vi "advanced_settings.vi"(0 "input cluster":T3) -> (1 "Output AFG resource name":refnum<k15>, 2 "Set?":bool)   [LabVIEW 2010]
uses:
  <vilib>/vision/Avi1.llb/AviRefnum.ctl
  <vilib>/userDefined/High Color/IMAQdx.ctl
panel:
  in  "Use Background Division Image Correction?":bool=TRUE
  in  "Aggregate Output?":bool
  in  "Number of Image Adaptation Bands":i32=10 step=1
  in  "stop":bool
  in  "OK Button":bool
  in  "AFG resource name":refnum<k15>="COM1"
  in  "Object Border":i32=20
  in  "Frames of Adaptation":i32=10
  in  "Bit Depth from Camera?":bool=TRUE
  in  "Image Bit Depth":u32=12
  in  "Adaptation Rate":i32=5 step=1
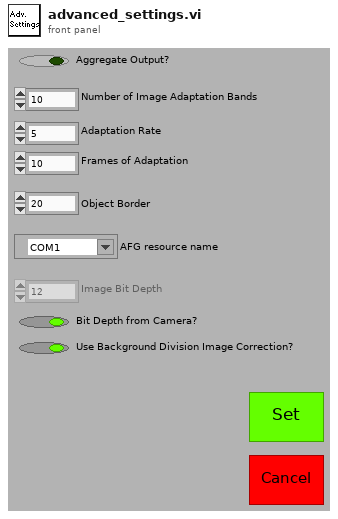
[diagram p1: front panel]
types:
  T1 = typedef "AviRefnum.ctl" = refnum<k1>
  T2 = typedef "IMAQdx.ctl" = refnum<k21>
  T3 = cluster{cluster{"Path":refnum<vi>, "Prefix":refnum<vi>, "Type of object to track":refnum<vi>, "Object Contrast (%)":refnum<vi>, "Fill Hysteresis (%)":refnum<vi>, "Maximum Object Size (pixels)":refnum<vi>, "Minimum Object Size (pixels)":refnum<vi>, "Object Size hysteresis (%)":refnum<vi>, "Image Binning":refnum<vi>, "Contour?":refnum<vi>, "Skeletonize?":refnum<vi>, "Frames of Adaptation":refnum<vi>, "Adaptation Rate":refnum<vi>, "Object Border":refnum<vi>, "Image Bit Depth":refnum<vi>, "Bit Depth from Camera?":refnum<vi>, "AFG resource name":refnum<vi>, "IMAQ Camera Interface Name":refnum<vi>, "Device auto-start delay (s)":refnum<vi>, "Number of Image Adaptation Bands":refnum<vi>, "Experiment Duration (s)":refnum<vi>, "Tap":refnum<vi>, "Tap Delay":refnum<vi>, "Tap Interval":refnum<vi>, "Tap Number":refnum<vi>, "Tap Stimulus Method":refnum<vi>, "Advanced Tap Settings":refnum<vi>, "Puff":refnum<vi>, "Puff Delay":refnum<vi>, "Puff Interval":refnum<vi>, "Puff Number":refnum<vi>, "Puff Stimulus Method":refnum<vi>, "Advanced Puff Settings":refnum<vi>, "Custom 1":refnum<vi>, "Custom 1 Delay":refnum<vi>, "Custom 1 Interval":refnum<vi>, "Custom 1 Number":refnum<vi>, "Custom 1 Stimulus Method":refnum<vi>, "Advanced Custom 1 Settings":refnum<vi>, "puff fraction of time between is active":refnum<vi>, "time between puff onset":refnum<vi>, "tap fraction of time between is active":refnum<vi>, "time between tap onset":refnum<vi>, "Tap Train Number":refnum<vi>, "custom 1 fraction of time between is active":refnum<vi>, "time between custom 1 onset":refnum<vi>, "Custom 2":refnum<vi>, "Custom 2 Delay":refnum<vi>, "Custom 2 Interval":refnum<vi>, "Custom 2 Number":refnum<vi>, "Custom 2 Stimulus Method":refnum<vi>, "Advanced Custom 2 Settings":refnum<vi>, "custom 2 fraction of time between is active":refnum<vi>, "time between custom 2 onset":refnum<vi>, "Save":refnum<vi>, "Load":refnum<vi>, "Raw Image Save Interval (s)":refnum<vi>, "Turn on output aggregation?":refnum<vi>, "Turn on Background division algorithm":refnum<vi>, "Turn on external triggering of camera":refnum<vi>}, cluster{"IMAQ Session Out":refnum<k11>, "Avi Refnum":T1, "Value":enum32{"IMAQ interface", "IMAQdx interface", "AVI file"}, "Value":T2, "Value":bool}}
  T4 = cluster{"Path":refnum<vi>, "Prefix":refnum<vi>, "Type of object to track":refnum<vi>, "Object Contrast (%)":refnum<vi>, "Fill Hysteresis (%)":refnum<vi>, "Maximum Object Size (pixels)":refnum<vi>, "Minimum Object Size (pixels)":refnum<vi>, "Object Size hysteresis (%)":refnum<vi>, "Image Binning":refnum<vi>, "Contour?":refnum<vi>, "Skeletonize?":refnum<vi>, "Frames of Adaptation":refnum<vi>, "Adaptation Rate":refnum<vi>, "Object Border":refnum<vi>, "Image Bit Depth":refnum<vi>, "Bit Depth from Camera?":refnum<vi>, "AFG resource name":refnum<vi>, "IMAQ Camera Interface Name":refnum<vi>, "Device auto-start delay (s)":refnum<vi>, "Number of Image Adaptation Bands":refnum<vi>, "Experiment Duration (s)":refnum<vi>, "Tap":refnum<vi>, "Tap Delay":refnum<vi>, "Tap Interval":refnum<vi>, "Tap Number":refnum<vi>, "Tap Stimulus Method":refnum<vi>, "Advanced Tap Settings":refnum<vi>, "Puff":refnum<vi>, "Puff Delay":refnum<vi>, "Puff Interval":refnum<vi>, "Puff Number":refnum<vi>, "Puff Stimulus Method":refnum<vi>, "Advanced Puff Settings":refnum<vi>, "Custom 1":refnum<vi>, "Custom 1 Delay":refnum<vi>, "Custom 1 Interval":refnum<vi>, "Custom 1 Number":refnum<vi>, "Custom 1 Stimulus Method":refnum<vi>, "Advanced Custom 1 Settings":refnum<vi>, "puff fraction of time between is active":refnum<vi>, "time between puff onset":refnum<vi>, "tap fraction of time between is active":refnum<vi>, "time between tap onset":refnum<vi>, "Tap Train Number":refnum<vi>, "custom 1 fraction of time between is active":refnum<vi>, "time between custom 1 onset":refnum<vi>, "Custom 2":refnum<vi>, "Custom 2 Delay":refnum<vi>, "Custom 2 Interval":refnum<vi>, "Custom 2 Number":refnum<vi>, "Custom 2 Stimulus Method":refnum<vi>, "Advanced Custom 2 Settings":refnum<vi>, "custom 2 fraction of time between is active":refnum<vi>, "time between custom 2 onset":refnum<vi>, "Save":refnum<vi>, "Load":refnum<vi>, "Raw Image Save Interval (s)":refnum<vi>, "Turn on output aggregation?":refnum<vi>, "Turn on Background division algorithm":refnum<vi>, "Turn on external triggering of camera":refnum<vi>}
  T5 = cluster{"IMAQ Session Out":refnum<k11>, "Avi Refnum":T1, "Value":enum32{"IMAQ interface", "IMAQdx interface", "AVI file"}, "Value":T2, "Value":bool}
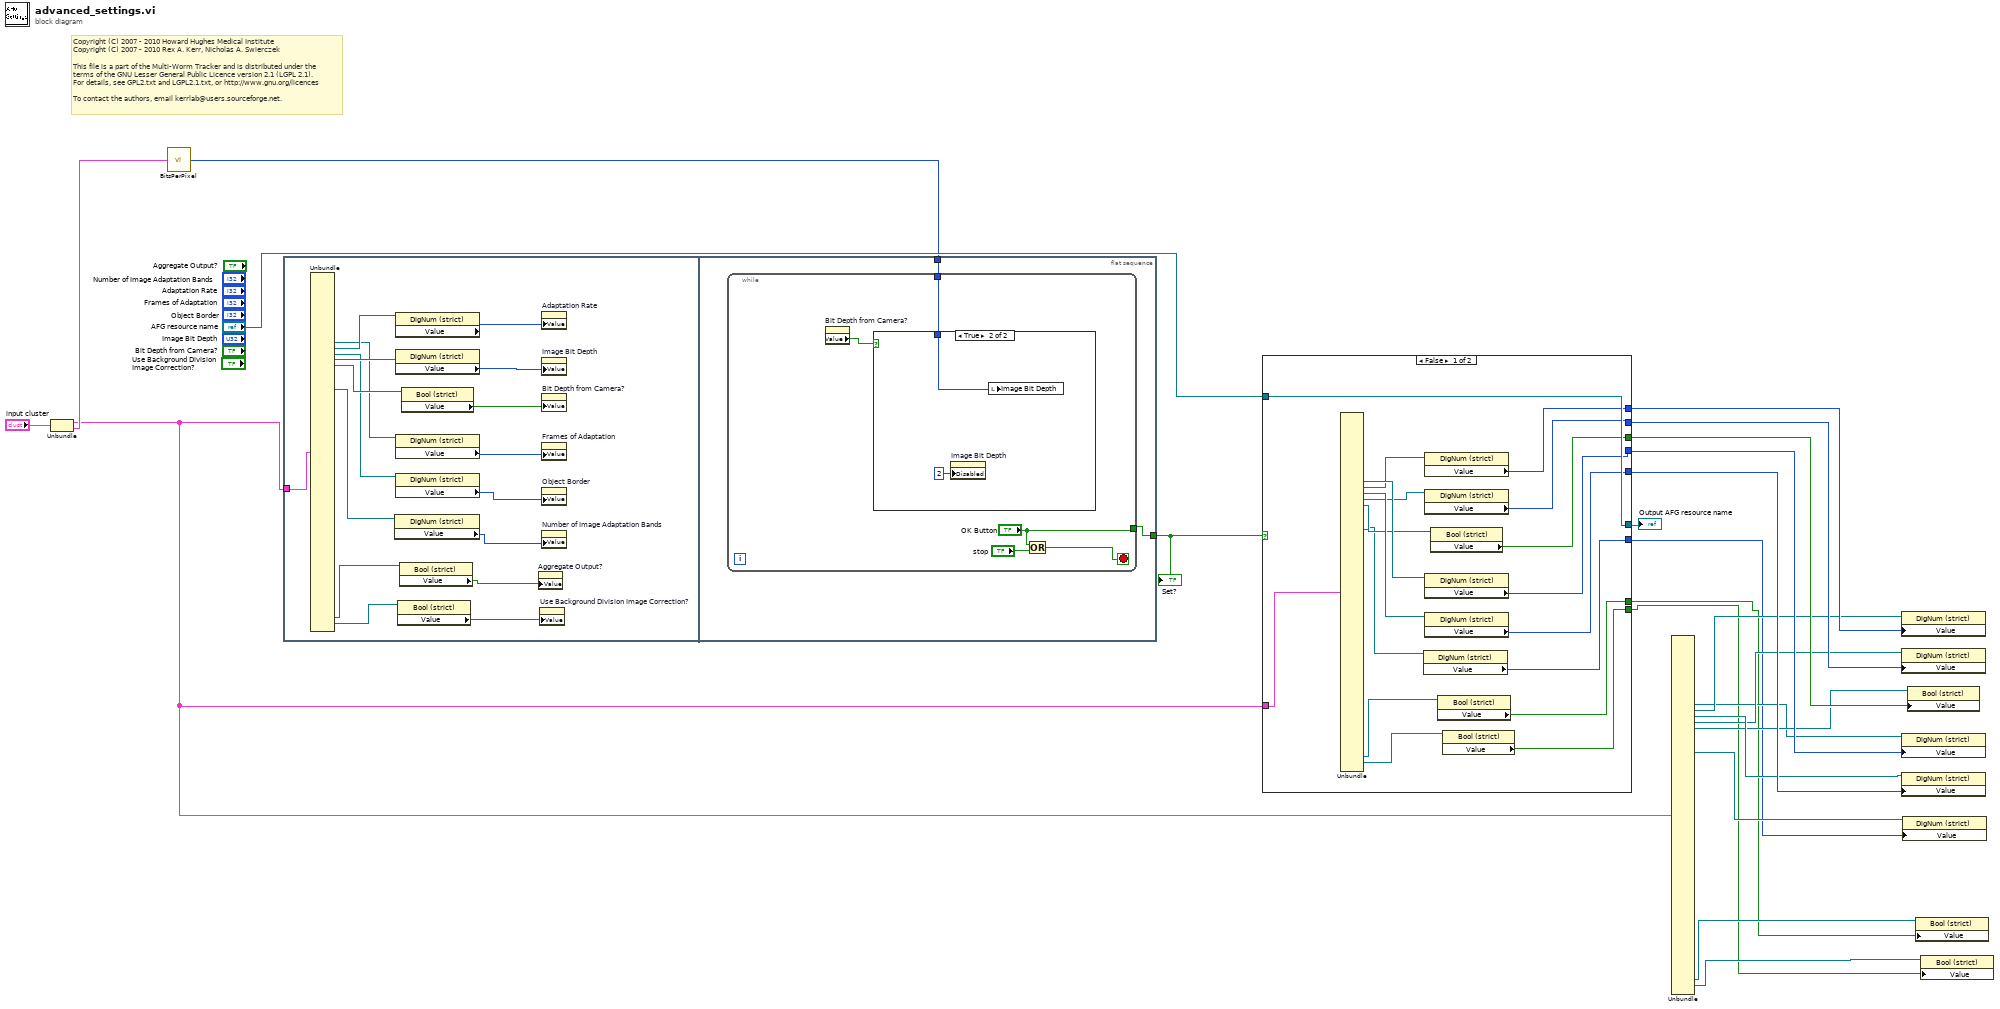
[diagram p0: block diagram]
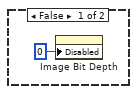
[diagram p2: hidden frame]
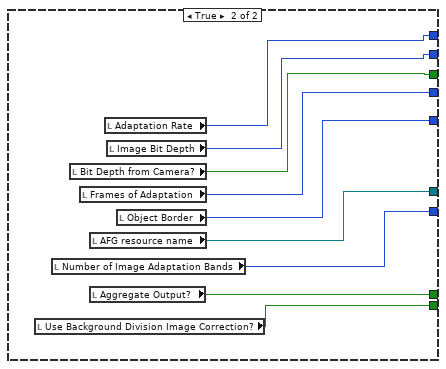
[diagram p3: hidden frame]
diagram:
  # "Copyright (C) 2007 - 2010 Howard Hughes Medical Institute\nCopyright (C) 2007 - 2010 Rex A. Kerr, Nicholas A. Swierczek\n \nThis file is a part of the Multi-Worm Tracker and is distributed under the\nterms of the GNU Lesser General Public Licence version 2.1 (LGPL 2.1).\nFor details, see GPL2.txt and LGPL2.1.txt, or http://www.gnu.org/licences\n \nTo contact the authors, email kerrlab@users.sourceforge.net."
  n1 = Unbundle("input cluster") -> (w6:T4, w7:T5)
  n2 = call "BitsPerPixel.vi"("camera cluster"=w7) -> ("BitsPerPixel"=w10:u32)
  n3 = flat-sequence {
    tunnel: w6 -> [w28]
    tunnel: [w42] -> w23
    tunnel: w10 -> [w41]
    frame #0 {
      n4 = Unbundle(w28) -> ("Frames of Adaptation"=w34:refnum<vi>, "Adaptation Rate"=w35:refnum<vi>, "Object Border"=w36:refnum<vi>, "Image Bit Depth"=w37:refnum<vi>, "Bit Depth from Camera?"=w38:refnum<vi>, "Number of Image Adaptation Bands"=w39:refnum<vi>, "Turn on output aggregation?"=w27:refnum<vi>, "Turn on Background division algorithm"=w25:refnum<vi>)  [unwired: 52 out]
      n5 = property class="DigNum (strict)"(reference=w39) -> ("Value"=w40:i32)  [unwired: 1 in, 2 out]
      n6 = property class="DigNum (strict)"(reference=w35) -> ("Value"=w29:i32)  [unwired: 1 in, 2 out]
      n7 = property class="DigNum (strict)"(reference=w37) -> ("Value"=w30:u32)  [unwired: 1 in, 2 out]
      n8 = property class="DigNum (strict)"(reference=w34) -> ("Value"=w32:i32)  [unwired: 1 in, 2 out]
      n9 = property class="DigNum (strict)"(reference=w36) -> ("Value"=w33:i32)  [unwired: 1 in, 2 out]
      n10 = property class="Bool (strict)"(reference=w25) -> ("Value"=w24:bool)  [unwired: 1 in, 2 out]
      n11 = property class="Bool (strict)"(reference=w27) -> ("Value"=w26:bool)  [unwired: 1 in, 2 out]
      n12 = property class="Bool (strict)"(reference=w38) -> ("Value"=w31:bool)  [unwired: 1 in, 2 out]
      n13 = property on="Aggregate Output?" class="Bool (strict)"("Value"=w26) -> ()  [unwired: 2 in, 2 out]
      n14 = property on="Use Background Division Image Correction?" class="Bool (strict)"("Value"=w24) -> ()  [unwired: 2 in, 2 out]
      n15 = property on="Adaptation Rate" class="DigNum (strict)"("Value"=w29) -> ()  [unwired: 2 in, 2 out]
      n16 = property on="Image Bit Depth" class="DigNum (strict)"("Value"=w30) -> ()  [unwired: 2 in, 2 out]
      n17 = property on="Bit Depth from Camera?" class="Bool (strict)"("Value"=w31) -> ()  [unwired: 2 in, 2 out]
      n18 = property on="Frames of Adaptation" class="DigNum (strict)"("Value"=w32) -> ()  [unwired: 2 in, 2 out]
      n19 = property on="Object Border" class="DigNum (strict)"("Value"=w33) -> ()  [unwired: 2 in, 2 out]
      n20 = property on="Number of Image Adaptation Bands" class="DigNum (strict)"("Value"=w40) -> ()  [unwired: 2 in, 2 out]
    }
    frame #1 {
      n21 = while {
        tunnel: ["OK Button"] -> w42
        tunnel: w41 -> [w43]
        stop <- w46 stop-if-true
        n22 = property on="Bit Depth from Camera?" class="Bool (strict)"() -> ("Value"=w44:bool)  [unwired: 2 in, 2 out]
        n23 = case shown="True" w44 {
          tunnel: w43 -> [_ w50]
          frame False {
            n24 = property on="Image Bit Depth" class="DigNum (strict)"("Disabled"=u8 0) -> ()  [unwired: 2 in, 2 out]
          }
          frame True {
            n25 = property on="Image Bit Depth" class="DigNum (strict)"("Disabled"=u8 2) -> ()  [unwired: 2 in, 2 out]
            n26 = local write "Image Bit Depth"(w50) -> ()
          }
        }
        n27 = Or(x="OK Button", y="stop") -> (x .or. y?=w46:bool)
      }
    }
  }
  n28 = case shown="False" w23 {
    tunnel: w6 -> [w68 _]
    tunnel: [w67 w77] -> w21
    tunnel: "AFG resource name" -> [w67 _]
    tunnel: [w66 w76] -> w20
    tunnel: [w65 w72] -> w19
    tunnel: [w64 w75] -> w18
    tunnel: [w63 w74] -> w17
    tunnel: [w62 w73] -> w16
    tunnel: [w56 w71] -> w8
    tunnel: [w53 w70] -> w4
    tunnel: [w51 w69] -> w2
    frame False {
      n29 = Unbundle(w68) -> ("Frames of Adaptation"=w61:refnum<vi>, "Adaptation Rate"=w60:refnum<vi>, "Object Border"=w59:refnum<vi>, "Image Bit Depth"=w58:refnum<vi>, "Bit Depth from Camera?"=w57:refnum<vi>, "Number of Image Adaptation Bands"=w55:refnum<vi>, "Turn on output aggregation?"=w54:refnum<vi>, "Turn on Background division algorithm"=w52:refnum<vi>)  [unwired: 52 out]
      n30 = property class="DigNum (strict)"(reference=w55) -> ("Value"=w56:i32)  [unwired: 1 in, 2 out]
      n31 = property class="DigNum (strict)"(reference=w60) -> ("Value"=w66:i32)  [unwired: 1 in, 2 out]
      n32 = property class="DigNum (strict)"(reference=w58) -> ("Value"=w65:u32)  [unwired: 1 in, 2 out]
      n33 = property class="DigNum (strict)"(reference=w61) -> ("Value"=w63:i32)  [unwired: 1 in, 2 out]
      n34 = property class="DigNum (strict)"(reference=w59) -> ("Value"=w62:i32)  [unwired: 1 in, 2 out]
      n35 = property class="Bool (strict)"(reference=w57) -> ("Value"=w64:bool)  [unwired: 1 in, 2 out]
      n36 = property class="Bool (strict)"(reference=w54) -> ("Value"=w53:bool)  [unwired: 1 in, 2 out]
      n37 = property class="Bool (strict)"(reference=w52) -> ("Value"=w51:bool)  [unwired: 1 in, 2 out]
    }
    frame True {
      n38 = local read "Use Background Division Image Correction?"() -> (w69:bool)
      n39 = local read "Number of Image Adaptation Bands"() -> (w71:i32)
      n40 = local read "Bit Depth from Camera?"() -> (w75:bool)
      n41 = local read "Frames of Adaptation"() -> (w74:i32)
      n42 = local read "AFG resource name"() -> (w77:refnum<k15>)
      n43 = local read "Aggregate Output?"() -> (w70:bool)
      n44 = local read "Adaptation Rate"() -> (w76:i32)
      n45 = local read "Image Bit Depth"() -> (w72:u32)
      n46 = local read "Object Border"() -> (w73:i32)
    }
  }
  "Output AFG resource name" <- w21
  n47 = Unbundle(w6) -> ("Frames of Adaptation"=w11:refnum<vi>, "Adaptation Rate"=w15:refnum<vi>, "Object Border"=w14:refnum<vi>, "Image Bit Depth"=w13:refnum<vi>, "Bit Depth from Camera?"=w12:refnum<vi>, "Number of Image Adaptation Bands"=w9:refnum<vi>, "Turn on output aggregation?"=w5:refnum<vi>, "Turn on Background division algorithm"=w3:refnum<vi>)  [unwired: 52 out]
  n48 = property class="DigNum (strict)"(reference=w15, "Value"=w20) -> ()  [unwired: 1 in, 2 out]
  n49 = property class="DigNum (strict)"(reference=w13, "Value"=w19) -> ()  [unwired: 1 in, 2 out]
  n50 = property class="DigNum (strict)"(reference=w11, "Value"=w17) -> ()  [unwired: 1 in, 2 out]
  n51 = property class="DigNum (strict)"(reference=w14, "Value"=w16) -> ()  [unwired: 1 in, 2 out]
  n52 = property class="DigNum (strict)"(reference=w9, "Value"=w8) -> ()  [unwired: 1 in, 2 out]
  n53 = property class="Bool (strict)"(reference=w12, "Value"=w18) -> ()  [unwired: 1 in, 2 out]
  n54 = property class="Bool (strict)"(reference=w5, "Value"=w4) -> ()  [unwired: 1 in, 2 out]
  n55 = property class="Bool (strict)"(reference=w3, "Value"=w2) -> ()  [unwired: 1 in, 2 out]
  "Set?" <- w23
